vi "protoWindow_1.0.vi"() -> ()   [LabVIEW 2014]
uses:
  common/crest/LabVIEW/LV14/libcommon-crest.lvlib
panel:
  in  "Dataset":path=path "/home/chaos/chaos_bundle/driver/powersupply/Labview/LV14/crest/datasets/btf_20150320_1052.dat"
  out "keys out":string
  out "values out":string
  out "parameters":string
  out "command":string
  out "element":string
  in  "Current Set [A]":dbl
  in  "set":bool
  in  "reset":bool
  in  "polaOpen":bool
  in  "polaPos":bool
  in  "polaNeg":bool
  out "fetch loop":i32
  out "index":i32
  in  "standby":bool
  in  "operational":bool
  in  "elementList":i32(listbox)
  in  "!CHAOS WAN url":string="192.168.150.91:8081"
  in  "enable window menu":bool
  in  "refreshConn":bool
  in  "set_to_saved":bool
  in  "local_load":bool
  in  "local_save":bool
  out "debug counter":i32
  # "ver. 1.0, build 20150320-1150"
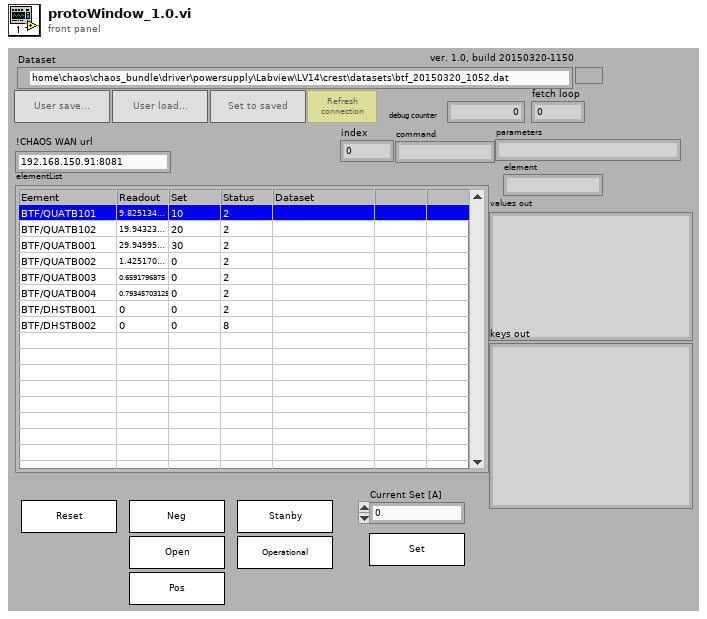
[diagram p1: front panel]
types:
  T1 = cluster{"numberOfElements":i32, "connectionHandle":u32, "selectedElement":i32}
  T2 = cluster{"currentReadout":string[], "currentSet":string[], "statusReadout":string[]}
  T3 = cluster{"elementNames":string[], "staAddresses":u32[], "dynAddddresses":u32[], "classIDs":i32[], "VME/ETH":bool[]}
  T4 = typedef "LVRectTypeDef.ctl" = cluster{"Left":i16, "Top":i16, "Right":i16, "Bottom":i16}
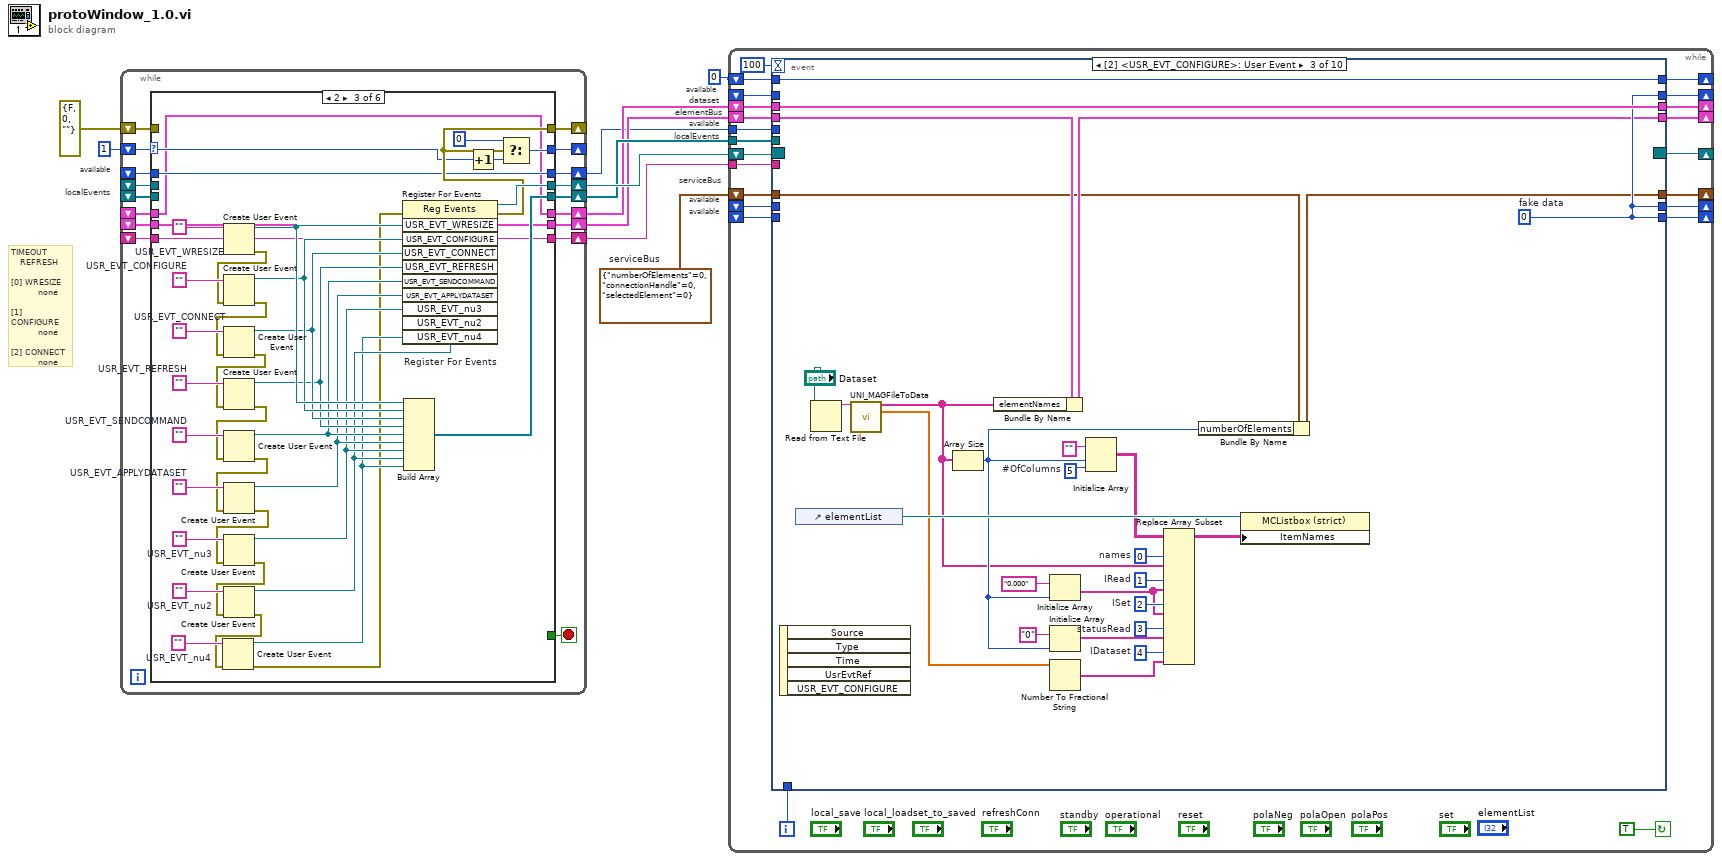
[diagram p0: block diagram]
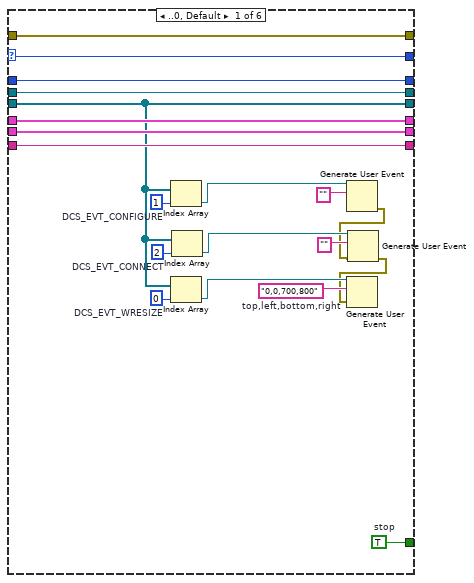
[diagram p2: hidden frame]
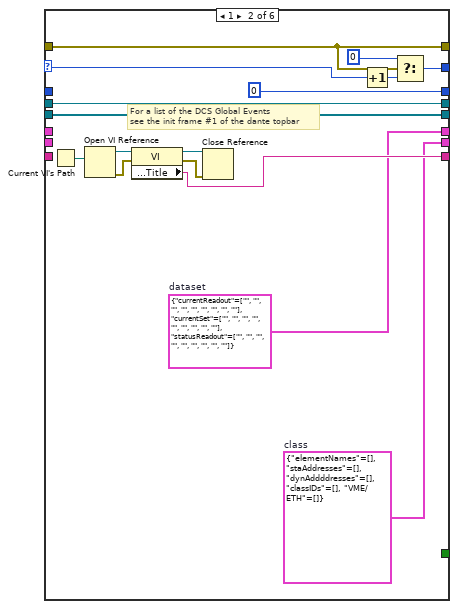
[diagram p3: hidden frame]
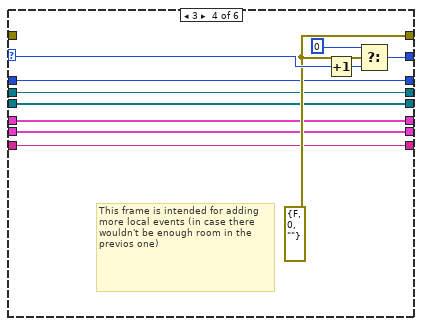
[diagram p4: hidden frame]
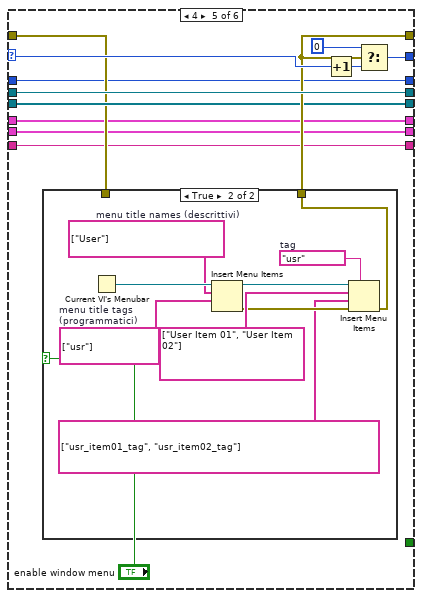
[diagram p5: hidden frame]
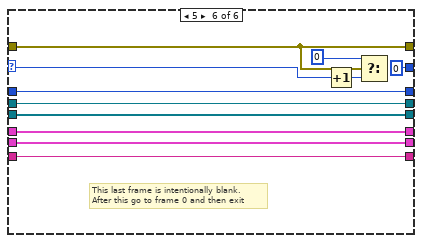
[diagram p7: hidden frame]
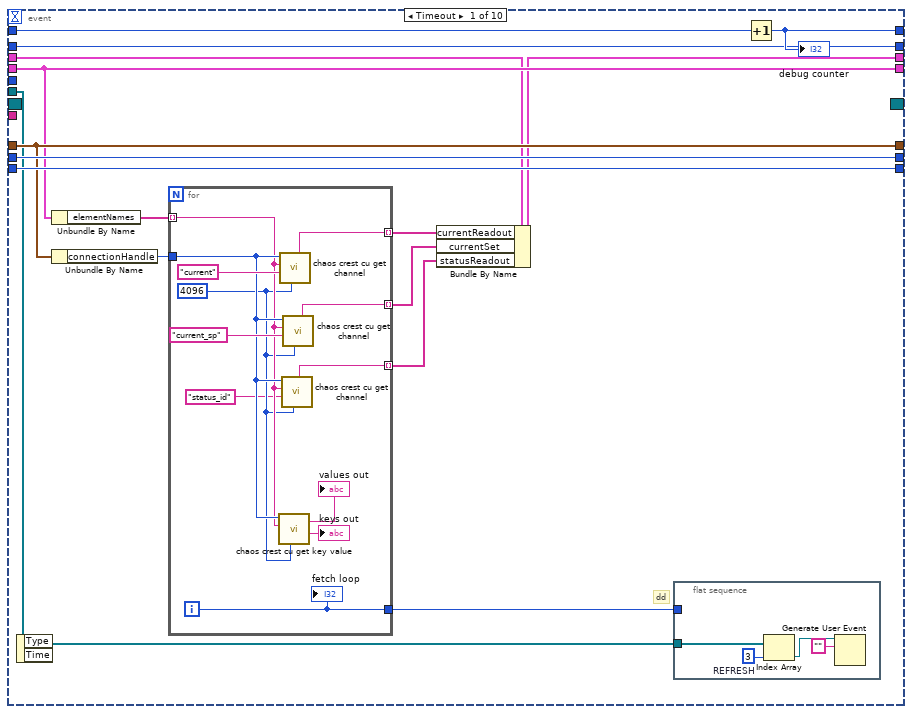
[diagram p8: hidden frame]
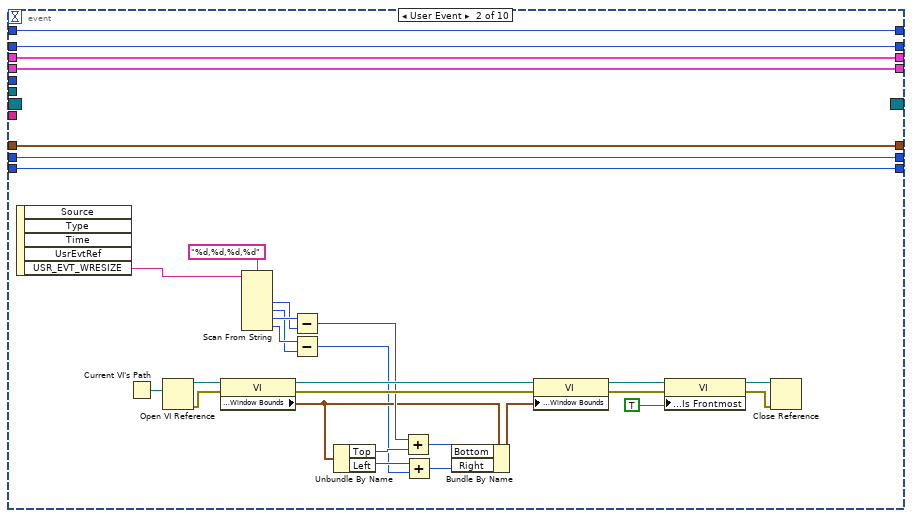
[diagram p9: hidden frame]
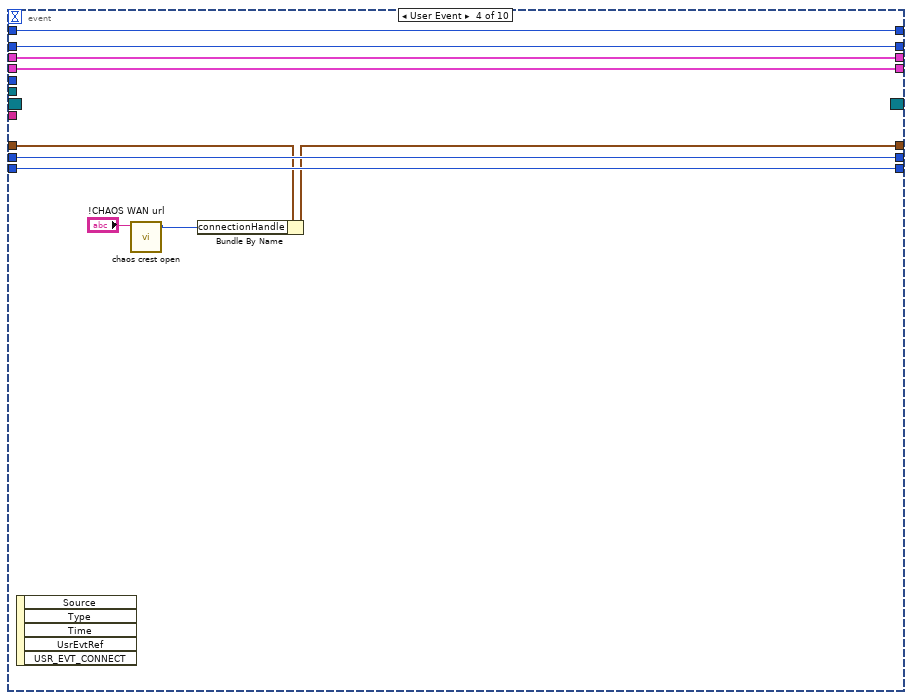
[diagram p10: hidden frame]
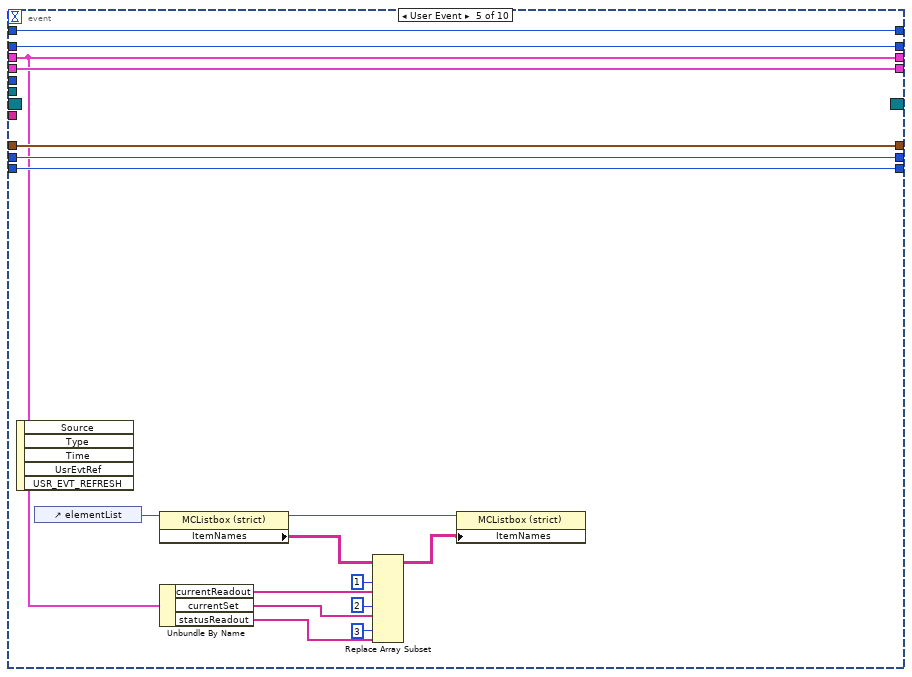
[diagram p11: hidden frame]
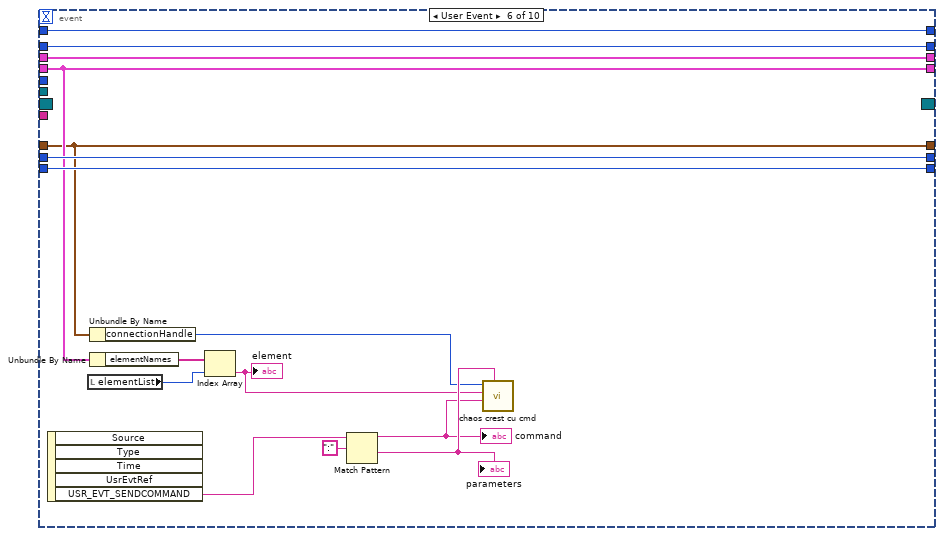
[diagram p12: hidden frame]
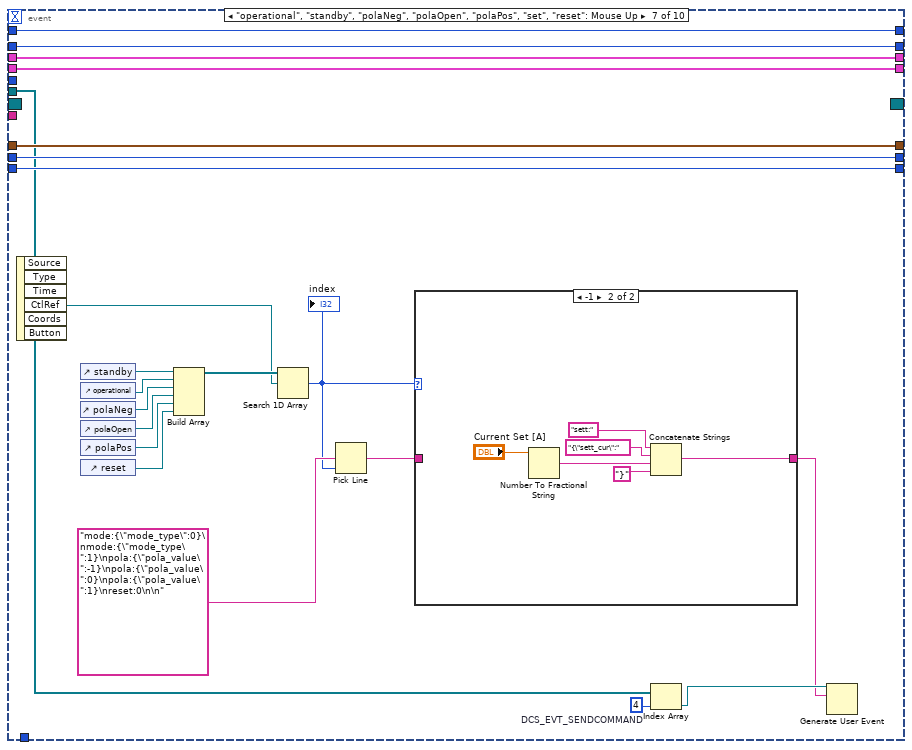
[diagram p13: hidden frame]
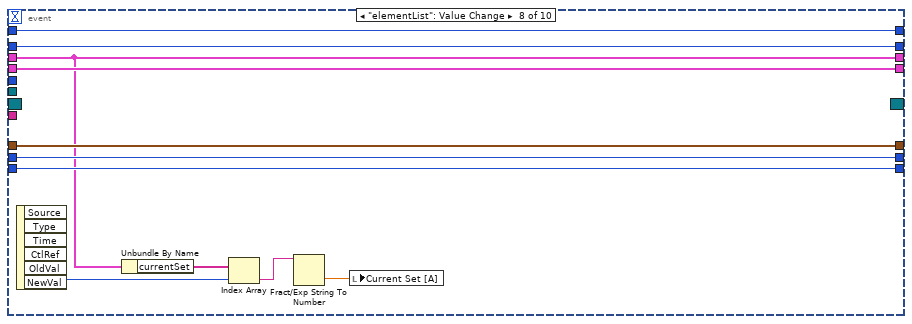
[diagram p15: hidden frame]
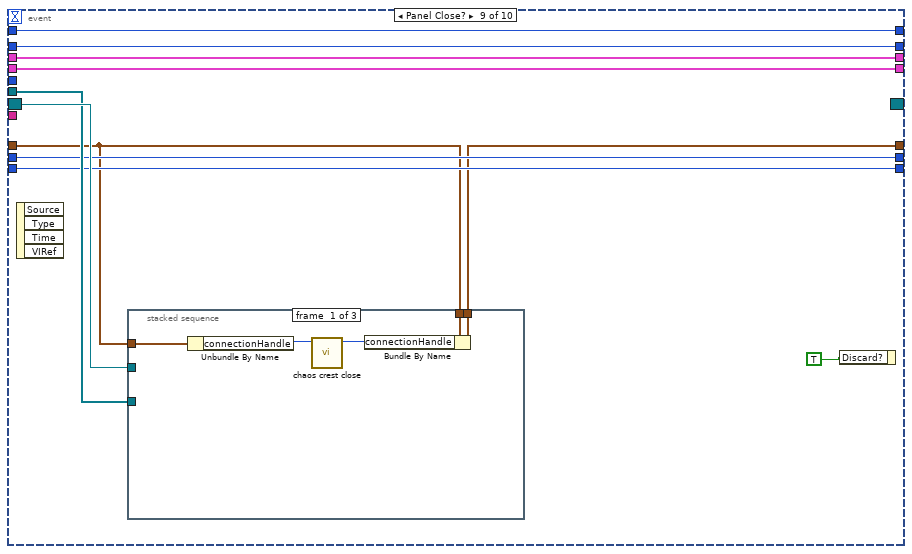
[diagram p16: hidden frame]
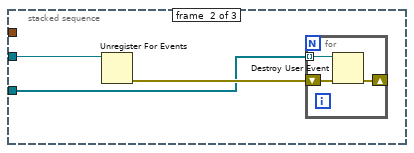
[diagram p17: hidden frame]
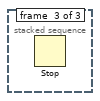
[diagram p18: hidden frame]
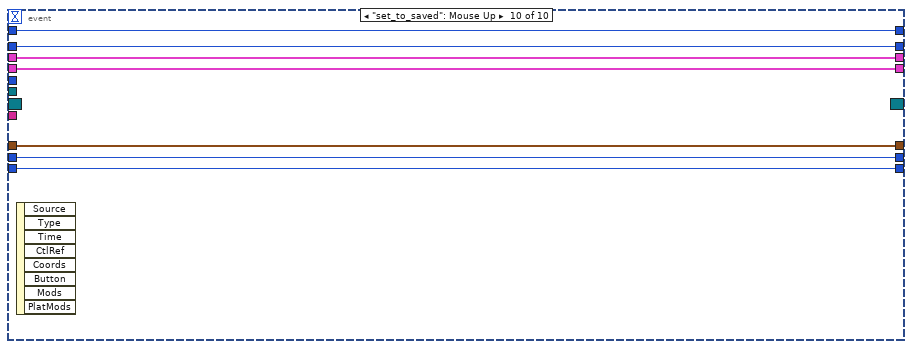
[diagram p19: hidden frame]
diagram:
  w4 = T1 {"numberOfElements"=0, "connectionHandle"=0, "selectedElement"=0}  # serviceBus
  # "available"
  # "serviceBus"
  # "TIMEOUT\n   REFRESH\n\n[0] WRESIZE\n         none\n\n[1] CONFIGURE\n         none\n\n[2] CONNECT\n         none"
  # "localEvents"
  # "available"
  # "localEvents"
  # "available"
  # "dataset"
  # "elementBus"
  # "available"
  # "available"
  n1 = while {
    shift-right: [w21] -> _
    shift-left: 1 -> [w24]
    shift-right: [w26] -> w8
    shift-left: _ -> [w23]
    shift-right: [w27] -> w6
    shift-left: _ -> [w22]
    shift-right: [w20] -> _
    shift-left: errorcluster {"status"=FALSE, "code"=0, "source"=""} ("error out") -> [w19]
    shift-right: [w18] -> w7
    shift-left: _ -> [w17]
    shift-right: [w16] -> w5
    shift-left: _ -> [w15]
    shift-right: [w14] -> w3
    shift-left: _ -> [w13]
    shift-right: [w12] -> w2
    shift-left: _ -> [w11]
    stop <- w25 stop-if-true
    n2 = case shown="2" w24 {
      tunnel: [w45 w48 w65 w104 w116 w140] -> w27
      tunnel: [w46 w63 w97 w106 w125 w143] -> w26
      selector: w24 -> [w43 w51 w92 w109 w121 w144]
      tunnel: [w47 _ _ _ _ _] -> w25
      tunnel: w23 -> [w46 w63 _ w106 w125 w143]
      tunnel: w22 -> [w45 _ w65 w104 w116 w140]
      tunnel: [w43 w53 w94 w110 w124 0 ("t")] -> w21
      tunnel: [w44 w52 w93 w108 w120 w137] -> w20
      tunnel: w19 -> [w44 w52 _ _ w117 w137]
      tunnel: [w28 w62 w91 w105 w119 w142] -> w18
      tunnel: w17 -> [w28 w62 _ w105 w119 w142]
      tunnel: [w42 w50 w64 w103 w115 w139] -> w16
      tunnel: w15 -> [w42 _ w64 w103 w115 w139]
      tunnel: [w38 0 w74 w107 w114 w138] -> w14
      tunnel: w13 -> [w38 _ w74 w107 w114 w138]
      tunnel: [w33 w56 w66 w102 w113 w136] -> w12
      tunnel: w11 -> [w33 _ w66 w102 w113 w136]
      frame ..0, Default {
        w32 = 1  # DCS_EVT_CONFIGURE
        w35 = 2  # DCS_EVT_CONNECT
        w39 = "0,0,700,800"  # top,left,bottom,right
        w41 = 0  # DCS_EVT_WRESIZE
        w47 = TRUE  # stop
        n3 = Index Array(array=w28, index=w32) -> (element=w31:refnum<user-event>)
        n4 = Index Array(array=w28, index=w41) -> (element=w40:refnum<user-event>)
        n5 = Index Array(array=w28, index=w35) -> (element=w36:refnum<user-event>)
        n6 = Generate User Event(user event=w31, event data cluster="" ("event data")) -> (error out=w29:errorcluster)  [unwired: 2 in, 1 out]
        n7 = Generate User Event(user event=w36, event data cluster="" ("event data"), error in=w29) -> (error out=w34:errorcluster)  [unwired: 1 in, 1 out]
        n8 = Generate User Event(user event=w40, event data cluster=w39, error in=w34) -> ()  [unwired: 1 in, 2 out]
      }
      frame 1 {
        w48 = T2 {"currentReadout"=["", "", "", "", "", "", "", "", ""], "currentSet"=["", "", "", "", "", "", "", "", ""], "statusReadout"=["", "", "", "", "", "", "", "", ""]}  # dataset
        w50 = T3 {"elementNames"=[], "staAddresses"=[], "dynAddddresses"=[], "classIDs"=[], "VME/ETH"=[]}  # class
        # "For a list of the DCS Global Events\nsee the init frame #1 of the dante topbar"
        n9 = Current VI's Path() -> (path=w57:path)
        n10 = Open VI Reference(vi path=w57) -> (vi reference=w60:refnum<vi>, error out=w58:errorcluster)  [unwired: 5 in]
        n11 = property class="VI"(reference=w60, error in=w58) -> (reference out=w61:refnum<vi>, error out=w59:errorcluster, "Front Panel Window:Title"=w56:string)
        n12 = Close Reference(reference=w61, error in (no error)=w59) -> ()  [unwired: 1 out]
        n13 = Increment(x=w51) -> (x+1=w55:i32)
        n14 = Select(t=0, s=w52, f=w55) -> (s? t:f=w53:i32)
      }
      frame 2 {
        w70 = ""  # USR_EVT_nu4
        w73 = ""  # USR_EVT_nu2
        w80 = ""  # USR_EVT_nu3
        w83 = ""  # USR_EVT_APPLYDATASET
        w86 = ""  # USR_EVT_SENDCOMMAND
        w88 = ""  # USR_EVT_REFRESH
        w90 = ""  # USR_EVT_CONNECT
        w98 = ""  # USR_EVT_CONFIGURE
        w101 = ""  # USR_EVT_WRESIZE
        n15 = Create User Event(user event datatype=w101) -> (user event=w100:refnum<user-event>, error out=w77:errorcluster)  [unwired: 1 in]
        n16 = Create User Event(user event datatype=w98, error in=w77) -> (user event=w99:refnum<user-event>, error out=w76:errorcluster)
        n17 = Create User Event(user event datatype=w90, error in=w76) -> (user event=w89:refnum<user-event>, error out=w75:errorcluster)
        n18 = Create User Event(user event datatype=w88, error in=w75) -> (user event=w87:refnum<user-event>, error out=w85:errorcluster)
        n19 = Create User Event(user event datatype=w86, error in=w85) -> (user event=w84:refnum<user-event>, error out=w82:errorcluster)
        n20 = Create User Event(user event datatype=w83, error in=w82) -> (user event=w81:refnum<user-event>, error out=w79:errorcluster)
        n21 = Create User Event(user event datatype=w80, error in=w79) -> (user event=w78:refnum<user-event>, error out=w72:errorcluster)
        n22 = Create User Event(user event datatype=w73, error in=w72) -> (user event=w71:refnum<user-event>, error out=w69:errorcluster)
        n23 = Create User Event(user event datatype=w70, error in=w69) -> (user event=w68:refnum<user-event>, error out=w67:errorcluster)
        n24 = register-events "Register For Events"(error in=w67, w100, w99, w89, w87, w84, w81, w78, w71, w68) -> (reference out=w97:refnum<event-registration>, error out=w93:errorcluster)  [unwired: 1 in]
        n25 = Build Array(w100, w99, w89, w87, w84, w81, w78, w71, w68) -> (w91:refnum<user-event>[])
        n26 = Increment(x=w92) -> (x+1=w96:i32)
        n27 = Select(t=0, s=w93, f=w96) -> (s? t:f=w94:i32)
      }
      frame 3 {
        w108 = errorcluster {"status"=FALSE, "code"=0, "source"=""} ("s")
        # "This frame is intended for adding more local events (in case there wouldn't be enough room in the previos one)"
        n28 = Increment(x=w109) -> (x+1=w112:i32)
        n29 = Select(t=0, s=w108, f=w112) -> (s? t:f=w110:i32)
      }
      frame 4 {
        n30 = case shown="True" "enable window menu" {
          tunnel: [w126 w127] -> w120
          tunnel: w117 -> [w126 _]
          frame False {
          }
          frame True {
            w134 = string[] ["User"]  # menu title names (descrittivi)
            w132 = "usr"  # tag
            w129 = string[] ["usr"]  # menu title tags (programmatici)
            n31 = Current VI's Menubar() -> (w135:refnum<k9>)
            n32 = Insert Menu Items(7:w129, 8:w134, 9:w135) -> (0:w130:errorcluster, 3:w131:refnum<k9>)  [unwired: 3 in, 1 out]
            n33 = Insert Menu Items(5:w132, 6:w130, 7:string[] ["usr_item01_tag", "usr_item02_tag"] ("item names"), 8:string[] ["User Item 01", "User Item 02"] ("item names"), 9:w131) -> (0:w127:errorcluster)  [unwired: 1 in, 2 out]
          }
        }
        n34 = Increment(x=w121) -> (x+1=w123:i32)
        n35 = Select(t=0, s=w120, f=w123) -> (s? t:f=w124:i32)
      }
      frame 5 {
        # "This last frame is intentionally blank.\nAfter this go to frame 0 and then exit"
        n36 = Increment(x=w144) -> (x+1=w146:i32)
        n37 = Select(t=0, s=w137, f=w146) -> ()  [unwired: 1 out]
      }
    }
  }
  n38 = while {
    shift-right: [w153] -> _
    shift-left: w6 -> [w154]
    shift-right: [w155] -> _
    shift-left: w5 -> [w156]
    shift-right: [w165] -> _
    shift-left: _ -> [w166]
    shift-right: [w167] -> _
    shift-left: _ -> [w164]
    shift-right: [w161] -> _
    shift-left: w8 -> [w163]
    tunnel: w7 -> [w162]
    shift-right: [w158] -> _
    shift-left: w4 -> [w159]
    tunnel: w3 -> [w157]
    tunnel: w2 -> [w152]
    shift-right: [w150] -> _
    shift-left: 0 ("debug counter") -> [w151]
    shift-right: [w148] -> _
    shift-left: _ -> [w149]
    i -> [w147]
    stop <- TRUE continue-if-true
    n39 = event shown="[2] <USR_EVT_CONFIGURE>: User Event" {
      selector: w163 -> [_ _ _ _ _ _ _ _ w350 _]
      dyn-events: [_ _ _ _ _ _ _ _ _ _] -> w161
      timeout: 100 -> [_ _ _ _ _ _ _ _ _ _]
      tunnel: [w180 w230 w256 w268 w284 w299 w321 w339 w347 w368] -> w167
      tunnel: w166 -> [w184 w231 _ w267 w285 w300 w322 w340 w348 w369]
      tunnel: [w184 w231 w256 w267 w285 w300 w322 w340 w348 w369] -> w165
      tunnel: w164 -> [w180 w230 _ w268 w284 w299 w321 w339 w347 w368]
      tunnel: w162 -> [w177 _ _ _ _ _ w305 _ w349 _]
      tunnel: w159 -> [w179 w225 w243 w261 w283 w288 w318 w338 w342 w363]
      tunnel: [w179 w225 w242 w260 w283 w288 w318 w338 w341 w363] -> w158
      tunnel: w157 -> [_ _ _ _ _ _ _ _ _ _]
      tunnel: w156 -> [w175 w228 w254 w262 w282 w295 w316 w333 w345 w366]
      tunnel: [w175 w228 w253 w262 w282 w295 w316 w333 w345 w366] -> w155
      tunnel: w154 -> [w173 w229 w258 w264 w274 w298 w320 w332 w346 w367]
      tunnel: [w172 w229 w258 w264 w274 w298 w320 w332 w346 w367] -> w153
      tunnel: w152 -> [_ _ _ _ _ _ _ _ _ _]
      tunnel: w151 -> [w183 w224 w257 w266 w281 w297 w319 w337 w344 w365]
      tunnel: [w182 w224 w257 w266 w281 w297 w319 w337 w344 w365] -> w150
      tunnel: [w181 w223 w256 w265 w280 w296 w317 w336 w343 w364] -> w148
      tunnel: w149 -> [w181 w223 _ w265 w280 w296 w317 w336 w343 w364]
      tunnel: w147 -> [_ _ _ _ _ _ _ _ _ _]
      event Timeout {
        # "dd"
        n40 = event-data() -> ()  [unwired: 1 in, 2 out]
        n41 = Unbundle By Name(w175) -> ("elementNames"=w174:string[])
        n42 = Unbundle By Name(w179) -> ("connectionHandle"=w178:u32)
        n43 = for {
          tunnel: w178 -> [w193]
          tunnel: [w199] -> w171 mode=indexing
          tunnel: [w198] -> w176
          tunnel: w174 -> [w192] mode=indexing
          tunnel: [w194] -> w170 mode=indexing
          tunnel: [w189] -> w169 mode=indexing
          i -> [w198]
          w191 = 4096 ("maxsize")
          n44 = call "chaos crest cu get key value.vi"("maxsize"=w191, "cuname"=w192, "handleConnection"=w193) -> ("keys out"=→"keys out":string, "values out"=→"values out":string)  [unwired: 5 in, 2 out]
          n45 = call "chaos crest cu get channel.vi"("maxsize"=w191, "channame"="current", "cuname"=w192, "handleConnection"=w193) -> ("value out"=w199:string)  [unwired: 6 in, 1 out]
          n46 = call "chaos crest cu get channel.vi"("maxsize"=w191, "channame"="status_id", "cuname"=w192, "handleConnection"=w193) -> ("value out"=w189:string)  [unwired: 6 in, 1 out]
          n47 = call "chaos crest cu get channel.vi"("maxsize"=w191, "channame"="current_sp", "cuname"=w192, "handleConnection"=w193) -> ("value out"=w194:string)  [unwired: 6 in, 1 out]
          "fetch loop" <- w198
        }
        n48 = Bundle By Name(cluster=w173, "currentReadout"=w171, "currentSet"=w170, "statusReadout"=w169) -> (w172:T2)
        n49 = flat-sequence {
          tunnel: w177 -> [w185]
          tunnel: w176 -> [_]
          frame #0 {
            w186 = 3  # REFRESH
            n50 = Index Array(array=w185, index=w186) -> (element=w187:refnum<user-event>)
            n51 = Generate User Event(user event=w187, event data cluster="" ("event data")) -> ()  [unwired: 2 in, 2 out]
          }
        }
        n52 = Increment(x=w183) -> (x+1=w182:i32)
        "debug counter" <- w182
      }
      event User Event {
        n53 = event-data() -> ("USR_EVT_WRESIZE"=w226:string)  [unwired: 1 in, 4 out]
        n54 = Current VI's Path() -> (path=w217:path)
        n55 = Open VI Reference(vi path=w217) -> (vi reference=w216:refnum<vi>, error out=w215:errorcluster)  [unwired: 5 in]
        n56 = property class="VI"(reference=w216, error in=w215) -> (reference out=w213:refnum<vi>, error out=w214:errorcluster, "Front Panel Window:Window Bounds"=w209:T4)
        n57 = Scan From String(format string="%d,%d,%d,%d", input string=w226) -> (output 1=w211:i32, output 2=w204:i32, output 3=w212:i32, output 4=w205:i32)  [unwired: 6 in, 3 out]
        n58 = Subtract(x=w212, y=w211) -> (x-y=w210:i32)
        n59 = Subtract(x=w205, y=w204) -> (x-y=w202:i32)
        n60 = Unbundle By Name(w209) -> ("Top"=w207:i16, "Left"=w203:i16)
        n61 = Add(x=w210, y=w207) -> (x+y=w206:i32)
        n62 = Add(x=w203, y=w202) -> (x+y=w201:i32)
        n63 = Bundle By Name(cluster=w209, "Bottom"=w206, "Right"=w201) -> (w208:T4)
        n64 = property class="VI"(reference=w213, error in=w214, "Front Panel Window:Window Bounds"=w208) -> (reference out=w218:refnum<vi>, error out=w219:errorcluster)
        n65 = property class="VI"(reference=w218, error in=w219, "Front Panel Window:Is Frontmost"=TRUE) -> (reference out=w221:refnum<vi>, error out=w222:errorcluster)
        n66 = Close Reference(reference=w221, error in (no error)=w222) -> ()  [unwired: 1 out]
      }
      event User Event {
        w234 = 4  # IDataset
        w235 = 3  # statusRead
        w245 = 2  # ISet
        w247 = 1  # IRead
        w241 = 5  # #OfColumns
        w252 = 0  # names
        w256 = 0  # fake data
        n67 = event-data() -> ()  [unwired: 1 in, 5 out]
        n68 = control-ref of="elementList"() -> (w250:refnum<vi>)
        n69 = Read from Text File(file (use dialog)="Dataset") -> (text=w255:string)  [unwired: 3 in, 3 out]
        n70 = call "UNI_MAGFileToData.vi"("spreadsheetData"=w255) -> ("names"=w237:string[], "settings"=w233:dbl[])  [unwired: 6 in, 7 out]
        n71 = Array Size(array=w237) -> (size(s)=w239:i32)
        n72 = Bundle By Name(cluster=w254, "elementNames"=w237) -> (w253:T3)
        n73 = Initialize Array("0.000" ("event data"), w239) -> (w244:string[])
        n74 = Initialize Array("0" ("event data"), w239) -> (w238:string[])
        n75 = Number To Fractional String(number=w233) -> (F-format string=w232:string[])  [unwired: 3 in]
        n76 = Initialize Array("" ("event data"), w239, w241) -> (w248:string[][])
        n77 = Replace Array Subset(array=w248, new element #1=w237, index (col) #1=w252, new element #2=w244, index (col) #2=w247, new element #3=w244, index (col) #3=w245, new element #4=w238, index (col) #4=w235, new element #5=w232, index (col) #5=w234) -> (w251:string[][])  [unwired: 5 in]
        n78 = Bundle By Name(cluster=w243, "numberOfElements"=w239) -> (w242:T1)
        n79 = property class="MCListbox (strict)"(reference=w250, "ItemNames"=w251) -> ()  [unwired: 1 in, 2 out]
      }
      event User Event {
        n80 = event-data() -> ()  [unwired: 1 in, 5 out]
        n81 = call "chaos crest open.vi"("chaoswanurl"="!CHAOS WAN url") -> ("handleConnection"=w259:u32)  [unwired: 10 in]
        n82 = Bundle By Name(cluster=w261, "connectionHandle"=w259) -> (w260:T1)
      }
      event User Event {
        n83 = event-data() -> ()  [unwired: 1 in, 5 out]
        n84 = control-ref of="elementList"() -> (w278:refnum<vi>)
        n85 = property class="MCListbox (strict)"(reference=w278) -> (reference out=w277:refnum<vi>, "ItemNames"=w276:string[][])  [unwired: 1 in, 1 out]
        n86 = Unbundle By Name(w274) -> ("currentReadout"=w273:string[], "currentSet"=w271:string[], "statusReadout"=w269:string[])
        n87 = Replace Array Subset(array=w276, new element #1=w273, index (col) #1=1 ("disabled index (col)"), new element #2=w271, index (col) #2=2 ("disabled index (col)"), new element #3=w269, index (col) #3=3 ("disabled index (col)")) -> (w275:string[][])  [unwired: 3 in]
        n88 = property class="MCListbox (strict)"(reference=w277, "ItemNames"=w275) -> ()  [unwired: 1 in, 2 out]
      }
      event User Event {
        n89 = event-data() -> ("USR_EVT_SENDCOMMAND"=w291:string)  [unwired: 1 in, 4 out]
        n90 = local read "elementList"() -> (w293:i32)
        n91 = Unbundle By Name(w288) -> ("connectionHandle"=w287:u32)
        n92 = Unbundle By Name(w295) -> ("elementNames"=w294:string[])
        n93 = Index Array(array=w294, index=w293) -> (element=w286:string)
        "element" <- w286
        n94 = Match Pattern(string=w291, regular expression=":") -> (before substring=w289:string, after substring=w290:string)  [unwired: 1 in, 2 out]
        "command" <- w289
        "parameters" <- w290
        n95 = call "chaos crest cu cmd.vi"("args"=w290, "cmd"=w289, "cuname"=w286, "handleConnection"=w287) -> ()  [unwired: 7 in, 1 out]
      }
      event "operational", "standby", "polaNeg", "polaOpen", "polaPos", "set", "reset": Mouse Up {
        w307 = 4  # DCS_EVT_SENDCOMMAND
        n96 = event-data() -> ("CtlRef"=w314:refnum<vi>)  [unwired: 1 in, 5 out]
        n97 = control-ref of="standby"() -> (w312:refnum<vi>)
        n98 = control-ref of="operational"() -> (w311:refnum<vi>)
        n99 = control-ref of="polaNeg"() -> (w310:refnum<vi>)
        n100 = control-ref of="polaOpen"() -> (w309:refnum<vi>)
        n101 = control-ref of="polaPos"() -> (w308:refnum<vi>)
        n102 = control-ref of="reset"() -> (w301:refnum<vi>)
        n103 = Build Array(w312, w311, w310, w309, w308, w301) -> (w315:refnum<vi>[])
        n104 = Search 1D Array(1D array=w315, element=w314) -> (index of element=w302:i32)  [unwired: 1 in]
        "index" <- w302
        n105 = Pick Line(multi-line string="mode:{\"mode_type\":0}\nmode:{\"mode_type\":1}\npola:{\"pola_value\":-1}\npola:{\"pola_value\":0}\npola:{\"pola_value\":1}\nreset:0\n\n", line index=w302) -> (output string=w304:string)  [unwired: 1 in]
        n106 = case shown="-1" w302 {
          tunnel: w304 -> [w323 _]
          tunnel: [w323 w325] -> w303
          frame Default {
          }
          frame -1 {
            n107 = Number To Fractional String(number="Current Set [A]") -> (F-format string=w327:string)  [unwired: 3 in]
            n108 = Concatenate Strings("sett:" ("cmd"), "{\"sett_cur\":", w327, "}" ("string")) -> (w325:string)
          }
        }
        n109 = Index Array(array=w305, index=w307) -> (element=w306:refnum<user-event>)
        n110 = Generate User Event(user event=w306, event data cluster=w303) -> ()  [unwired: 2 in, 2 out]
      }
      event "elementList": Value Change {
        n111 = event-data() -> ("NewVal"=w334:i32)  [unwired: 1 in, 5 out]
        n112 = Unbundle By Name(w332) -> ("currentSet"=w335:string[])
        n113 = Index Array(array=w335, index=w334) -> (element=w331:string)
        n114 = Fract/Exp String To Number(string=w331) -> (number=w330:dbl)  [unwired: 3 in, 1 out]
        n115 = local write "Current Set [A]"(w330) -> ()
      }
      event Panel Close? {
        n116 = event-data() -> ()  [unwired: 1 in, 4 out]
        n117 = stacked-sequence {
          tunnel: w350 -> [_ w358 _]
          tunnel: w349 -> [_ w357 _]
          tunnel: w342 -> [w355 _ _]
          tunnel: w342 -> [w354 _ _]
          tunnel: [w353 _ _] -> w341
          frame #0 {
            n118 = Unbundle By Name(w355) -> ("connectionHandle"=w356:u32)
            n119 = call "chaos crest close.vi"("connectionHandle"=w356) -> ("connectionHandle out"=w352:u32)  [unwired: 9 in, 1 out]
            n120 = Bundle By Name(cluster=w354, "connectionHandle"=w352) -> (w353:T1)
          }
          frame #1 {
            n121 = Unregister For Events(event registration refnum=w358) -> (error out=w359:errorcluster)  [unwired: 1 in]
            n122 = for {
              tunnel: w357 -> [w362] mode=indexing
              shift-right: [w360] -> _
              shift-left: w359 -> [w361]
              n123 = Destroy User Event(user event=w362, error in=w361) -> (error out=w360:errorcluster)
            }
          }
          frame #2 {
            n124 = Stop() -> ()  [unwired: 1 in]
          }
        }
        n125 = event-data("Discard?"=TRUE) -> ()  [unwired: 1 in, 1 out]
      }
      event "set_to_saved": Mouse Up {
        n126 = event-data() -> ()  [unwired: 1 in, 8 out]
      }
    }
  }
